vi "IndexUpdate.vi"(0 "ScanStepIn":i32[](array[numeric]), 1 "ScanSizes":i32[](array[numeric])) -> (2 "Done":bool, 3 "Update?":bool[](array[boolean]), 4 "ScanStepOut":i32[](array[numeric]))   [LabVIEW 2017]
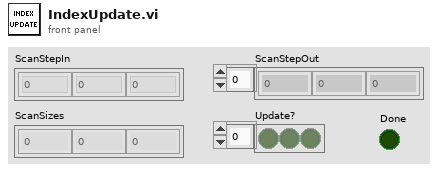
[diagram p1: front panel]
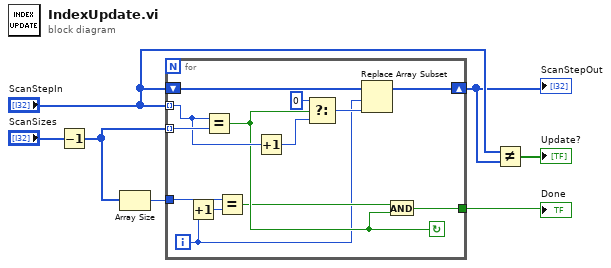
[diagram p0: block diagram]
diagram:
  n1 = Decrement(x="ScanSizes") -> (x-1=w4:i32[])
  n2 = Array Size(array=w4) -> (size(s)=w7:i32)
  n3 = for {
    tunnel: "ScanStepIn" -> [w19] mode=indexing
    tunnel: w4 -> [w20] mode=indexing
    shift-right: [w16] -> w2
    shift-left: "ScanStepIn" -> [w18]
    tunnel: w7 -> [w14]
    tunnel: [w12] -> w6
    i -> [w8]
    stop <- w15 continue-if-true
    n4 = Increment(x=w8) -> (x+1=w9:i32)
    n5 = Equal?(x=w19, y=w20) -> (x = y?=w15:bool)
    n6 = Equal?(x=w14, y=w9) -> (x = y?=w13:bool)
    n7 = Increment(x=w19) -> (x+1=w10:i32)
    n8 = Select(t=0 ("f"), s=w15, f=w10) -> (s? t:f=w17:i32)
    n9 = Replace Array Subset(array=w18, new element=w17, index=w8) -> (w16:i32[])
    n10 = And(x=w13, y=w15) -> (x .and. y?=w12:bool)
  }
  "Done" <- w6
  "ScanStepOut" <- w2
  n11 = Not Equal?(x="ScanStepIn", y=w2) -> (x != y?=→"Update?":bool[])
